vi "RM.Manager UI.vi"(8 "error in (no error)":errorcluster, 11 "Node Ptr":T1 format="%.0x") -> ()   [LabVIEW 2016, in "FPGA Resource Manager.lvlib"]
uses:
  FPGA Resource Manager.lvlib
  <vilib>/NI Veristand/Custom Device API/Custom Device Item Ref.ctl
  <vilib>/NI Veristand/Custom Device API/Custom Device API.lvlib
panel:
  in  "Tree":string(tree)
  in  "Listbox":i32(listbox)
  in  "button_done":bool
  # "FPGA Resource Manager"
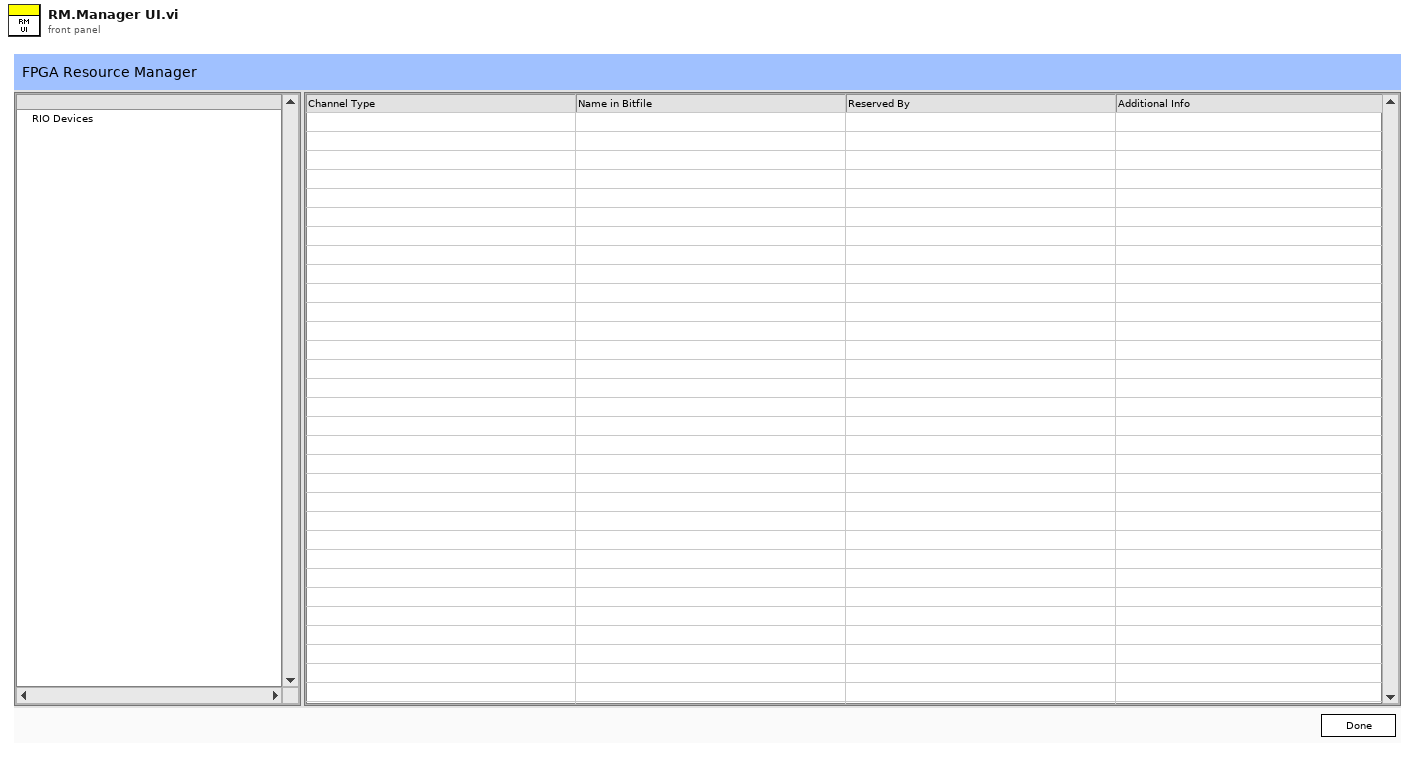
[diagram p1: front panel]
types:
  T1 = typedef "Custom Device API.lvlib/Custom Device Item Ref.ctl" = u64
  T2 = typedef "FPGA Resource Manager.lvlib/RM.serverInfo.ctl" = cluster{"name":string, "guid":string, "cd node ref":T1, "database":variant}
  T3 = cluster{"Left Cell String":string, "Child Text":string[], "Child Tag":string, "Item Indent":i32, "Child Only?":bool, "Glyph Index":i32}[]
  T4 = typedef "FPGA Resource Manager.lvlib/RM.clientInfo.ctl" = cluster{"Name":string, "GUID":string, "CD Ref":T1}
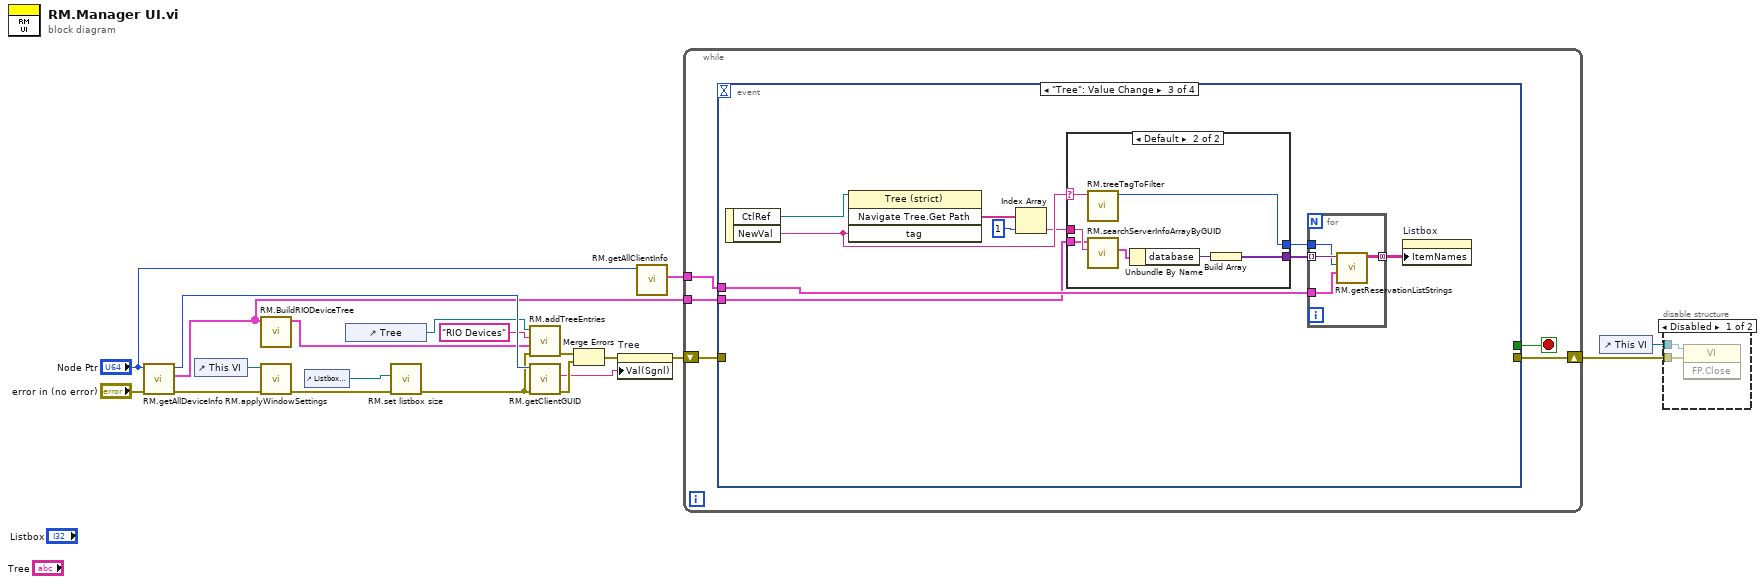
[diagram p0: block diagram]
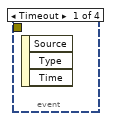
[diagram p3: hidden frame]
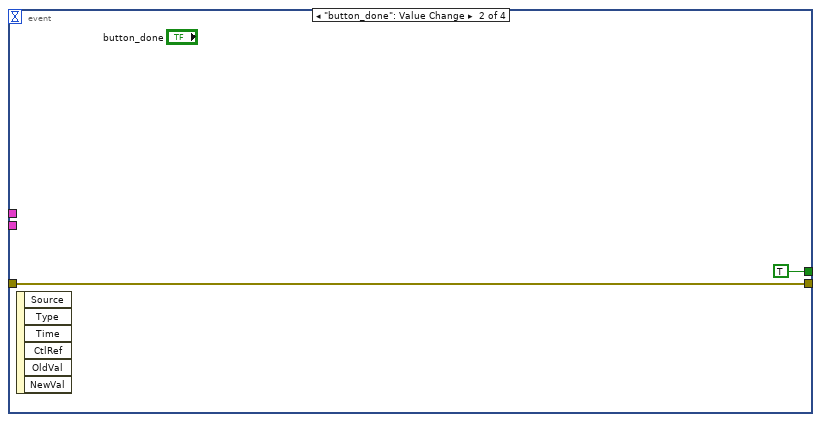
[diagram p4: hidden frame]
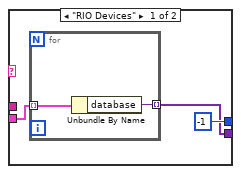
[diagram p5: hidden frame]
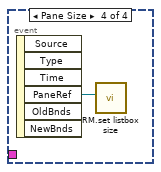
[diagram p6: hidden frame]
diagram:
  n1 = call "RM.getAllDeviceInfo.vi"("error in"="error in (no error)", "Item Ref in"="Node Ptr") -> ("error out"=w7:errorcluster, "deviceInfo array"=w1:T2[], "Item Ref out"=w17:T1)  [unwired: 7 in]
  n2 = control-ref of="This VI"() -> (w12:refnum<vi>)
  n3 = call "RM.BuildRIODeviceTree.vi"("deviceInfo array"=w1) -> ("RIO Device Tree Entries"=w10:T3)  [unwired: 10 in]
  n4 = call "RM.applyWindowSettings.vi"("error in (no error)"=w7, "VI reference"=w12) -> ("error out"=w4:errorcluster)  [unwired: 9 in]
  n5 = control-ref of="Listbox Pane"() -> (w18:refnum<vi>)
  n6 = control-ref of="Tree"() -> (w11:refnum<vi>)
  n7 = call "RM.set listbox size.vi"("error in (no error)"=w4, "Pane Refnum"=w18) -> ("error out"=w3:errorcluster)  [unwired: 9 in]
  n8 = call "RM.addTreeEntries.vi"("error in (no error)"=w3, "Entries"=w10, "Group Name"="RIO Devices", "TreeControl in"=w11) -> ("error out"=w16:errorcluster)  [unwired: 7 in]
  n9 = call "RM.getClientGUID.vi"("error in (no error)"=w3, "Item Ref in"=w17) -> ("error out"=w5:errorcluster, "ClientGUID"=w2:string)  [unwired: 6 in, 2 out]
  n10 = Merge Errors(w16, w5) -> (w6:errorcluster)
  n11 = property on="Tree" class="Tree (strict)"(error in=w6, "Val(Sgnl)"=w2) -> (error out=w15:errorcluster)  [unwired: 1 in, 1 out]
  n12 = call "RM.getAllClientInfo.vi"("Item Ref in"="Node Ptr") -> ("ClientInfo Array"=w13:T4[])  [unwired: 8 in, 2 out]
  n13 = while {
    shift-right: [w23] -> w19
    shift-left: w15 -> [w24]
    tunnel: w13 -> [w22]
    tunnel: w1 -> [w21]
    stop <- w25 stop-if-true
    n14 = event shown="[2] \"Tree\": Value Change" {
      selector: _ -> [_ _ _ _]
      dyn-events: _ -> [_ _ _ _]
      timeout: _ -> [_ _ _ _]
      tunnel: [_ TRUE _ _] -> w25
      tunnel: w24 -> [_ w26 _ _]
      tunnel: [_ w26 _ _] -> w23
      tunnel: w22 -> [_ _ w29 _]
      tunnel: w21 -> [_ _ w28 _]
      event Timeout {
        n15 = event-data() -> ()  [unwired: 1 in, 3 out]
      }
      event "button_done": Value Change {
        n16 = event-data() -> ()  [unwired: 1 in, 6 out]
      }
      event "Tree": Value Change {
        n17 = event-data() -> ("CtlRef"=w34:refnum<vi>, "NewVal"=w32:string)  [unwired: 1 in]
        n18 = invoke class="Tree (strict)" method="Navigate Tree.Get Path"(reference=w34, "tag"=w32) -> ("Navigate Tree:Get Path"=w36:string[])  [unwired: 2 in, 3 out]
        n19 = Index Array(array=w36, index=1) -> (element=w30:string)
        n20 = case shown="Default" w32 {
          selector: w32 -> [_ w53]
          tunnel: [w42 w51] -> w37
          tunnel: [-1 w52] -> w33
          tunnel: w30 -> [_ w50]
          tunnel: w28 -> [w43 w49]
          frame "RIO Devices" {
            n21 = for {
              tunnel: w43 -> [w46] mode=indexing
              tunnel: [w45] -> w42 mode=indexing
              n22 = Unbundle By Name(w46) -> ("database"=w45:variant)
            }
          }
          frame Default {
            n23 = call "RM.treeTagToFilter.vi"("tree tag"=w53) -> ("filter type"=w52:i32)  [unwired: 10 in]
            n24 = call "RM.searchServerInfoArrayByGUID.vi"("selected deviceGUID"=w50, "serverInfo array in"=w49) -> ("serverInfo"=w47:T2)  [unwired: 6 in, 3 out]
            n25 = Unbundle By Name(w47) -> ("database"=w48:variant)
            n26 = Build Array(w48) -> (w51:variant[])
          }
        }
        n27 = for {
          tunnel: w37 -> [w41] mode=indexing
          tunnel: [w39] -> w35 mode=concatenating
          tunnel: w33 -> [w40]
          tunnel: w29 -> [w38]
          n28 = call "RM.getReservationListStrings.vi"("ClientInfo Array"=w38, "type filter"=w40, "reservation db"=w41) -> ("Reservation List Array"=w39:string[][])  [unwired: 7 in, 1 out]
        }
        n29 = property on="Listbox" class="MCListbox (strict)"("ItemNames"=w35) -> ()  [unwired: 2 in, 2 out]
      }
      event Pane Size {
        n30 = event-data() -> ("PaneRef"=w54:refnum<vi>)  [unwired: 1 in, 5 out]
        n31 = call "RM.set listbox size.vi"("Pane Refnum"=w54) -> ()  [unwired: 10 in, 1 out]
      }
    }
  }
  n32 = control-ref of="This VI"() -> (w20:refnum<vi>)
  n33 = disable-structure shown="Disabled" {
    disable-tunnel: w20 -> [w56 _]
    disable-tunnel: w19 -> [w55 _]
    frame Disabled {
      n34 = invoke class="VI" method="FP.Close"(reference=w56, error in=w55) -> ()  [unwired: 1 in, 3 out]
    }
    frame Enabled {
    }
  }
